vi "creat new file.vi"(7 "file name":string, 8 "error in (no error)":errorcluster caption="错误输入（无错误）", 11 "path":path) -> (0 "error out":errorcluster, 2 "file or folder exists?":bool caption="文件或文件夹存在？", 3 "created path":path)   [LabVIEW 2018]
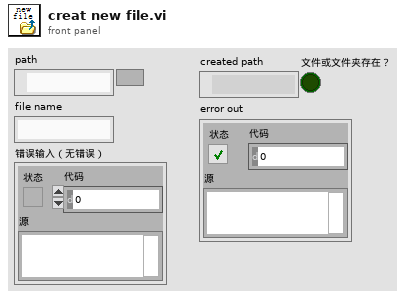
[diagram p1: front panel]
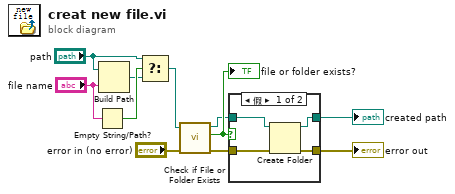
[diagram p0: block diagram]
diagram:
  n1 = Empty String/Path?(string/path="file name") -> (empty?=w5:bool)
  n2 = Build Path(base path="path", name or relative path="file name") -> (appended path=w3:path)
  n3 = Select(t="path", s=w5, f=w3) -> (s? t:f=w4:path)
  n4 = call <vilib>:"Check if File or Folder Exists.vi"("error in (no error)"="error in (no error)", "path"=w4) -> ("error out"=w7:errorcluster, "file or folder exists?"=w10:bool, "dup path"=w9:path)  [unwired: 7 in]
  "file or folder exists?" <- w10
  n5 = case shown="假" w10 {
    tunnel: [w12 w17] -> w8
    tunnel: w9 -> [w15 w17]
    tunnel: [w13 w16] -> w6
    tunnel: w7 -> [w14 w16]
    frame False {
      n6 = Create Folder(path (use dialog)=w15, error in=w14) -> (created path=w12:path, error out=w13:errorcluster)  [unwired: 1 in, 1 out]
    }
    frame True {
    }
  }
  "created path" <- w8
  "error out" <- w6
